vi "FF, Acceptance Criteria.vi"(8 "error in":errorcluster, 9 "n rows":i32=10, 10 "test case":T1, 11 "Tbl Refnum":refnum<vi>) -> (0 "error out":errorcluster, 3 "Tbl Refnum out":refnum<vi>)   [LabVIEW 2010]
doc: "This function transfers a single Compare Data Test (CDT) record to the current TestStand sequence step."
uses:
  Active Output Test Cases.ctl
panel:
  in  "Initialize Table":bool
  out "import error":errorcluster caption="error out"
  in  "Excel Clipboard to Import":string="TRS1763\tStimulus Phase Amplitude\t\t-5.170\t-4.830\tmA\tGELE\t%.3f\t%.3f\tTC1\nTRS1762\tStimulus Phase Pulse Width\t\t7.52\t16.48\tus\tGELE\t%.2f\t%.2f\tTC1\nTRS1761\tActive Interphase Delay\t\t13.0\t27.0\tus\tGELE\t%.1f\t%.1f\tTC1\nTRS1760\tActive Recovery Phase Amplitude\t\t4.830\t5.170\tmA\tGELE\t%.3f\t%.3f\tTC1\nTRS1759\tActive Recovery Phase Pulse Width\t\t7.5\t16.5\tus\tGELE\t%.1f\t%.1f\tTC1\nTRS1758\tFrequency\t\t1930.0\t2070.0\tHz\tGELE\t%.1f\t%.1f\tTC1\nTRS1757\tPulse Period Jitter (RMS)\t\t-2.500\t2.500\tus\tGELE\t%.1f\t%.1f\tTC1\nTRS1770\tStimulus Phase Amplitude\t\t-0.125\t0.085\tmA\tGELE\t%.3f\t%.3f\tTC2\nTRS1769\tStimulus Phase Pulse Width\t\t1436.0\t1564.0\tus\tGELE\t%.1f\t%.1f\tTC2\nTRS1768\tActive Interphase Delay\t\t233.0\t247.0\tus\tGELE\t%.1f\t%.1f\tTC2\nTRS1767\tActive Recovery Phase Amplitude\t\t-0.085\t0.125\tmA\tGELE\t%.3f\t%.3f\tTC2\nTRS1766\tActive Recovery Phase Pulse Width\t\t1436.0\t1564.0\tus\tGELE\t%.1f\t%.1f\tTC2\nTRS1765\tFrequency\t\t21.230\t22.770\tHz\tGELE\t%.3f\t%.3f\tTC2\nTRS1764\tPulse Period Jitter (RMS)\t\t-227.273\t227.273\tus\tGELE\t%.1f\t%.1f\tTC2\nTRS1777\tStimulus Phase Amplitude\t\t-15.320\t-14.680\tmA\tGELE\t%.3f\t%.3f\tTC3\nTRS1776\tStimulus Phase Pulse Width\t\t380.000\t420.000\tus\tGELE\t%.1f\t%.1f\tTC3\nTRS1775\tActive Interphase Delay\t\t93.0\t107.0\tus\tGELE\t%.1f\t%.1f\tTC3\nTRS1774\tActive Recovery Phase Amplitude\t\t14.680\t15.320\tmA\tGELE\t%.3f\t%.3f\tTC3\nTRS1773\tActive Recovery Phase Pulse Width\t\t380.00\t420.00\tus\tGELE\t%.1f\t%.1f\tTC3\nTRS1772\tFrequency\t\t1.930\t2.070\tHz\tGELE\t%.3f\t%.3f\tTC3\nTRS1771\tPulse Period Jitter (RMS)\t\t-2500.0\t2500.0\tus\tGELE\t%.1f\t%.1f\tTC3\nTRS1784\tStimulus Phase Amplitude\t\t2.850\t3.150\tmA\tGELE\t%.3f\t%.3f\tTC4\nTRS1783\tStimulus Phase Pulse Width\t\t1436.0\t1564.0\tus\tGELE\t%.1f\t%.1f\tTC4\nTRS1782\tActive Interphase Delay\t\t233.0\t247.0\tus\tGELE\t%.1f\t%.1f\tTC4\nTRS1781\tActive Recovery Phase Amplitude\t\t-0.726\t-0.474\tmA\tGELE\t%.3f\t%.3f\tTC4\nTRS1780\tActive Recovery Phase Pulse Width\t\t7180.0\t7820.0\tus\tGELE\t%.1f\t%.1f\tTC4\nTRS1779\tFrequency\t\t48.3\t51.8\tHz\tGELE\t%.1f\t%.1f\tTC4\nTRS1778\tPulse Period Jitter (RMS)\t\t-100.0\t100.0\tus\tGELE\t%.1f\t%.1f\tTC4\nTRS1791\tStimulus Phase Amplitude\t\t-0.085\t0.125\tmA\tGELE\t%.3f\t%.3f\tTC5\nTRS1790\tStimulus Phase Pulse Width\t\t1436.0\t1564.0\tus\tGELE\t%.1f\t%.1f\tTC5\nTRS1789\tActive Interphase Delay\t\t233.0\t247.0\tus\tGELE\t%.1f\t%.1f\tTC5\nTRS1788\tActive Recovery Phase Amplitude\t\t-0.125\t0.085\tmA\tGELE\t%.3f\t%.3f\tTC5\nTRS1787\tActive Recovery Phase Pulse Width\t\t1436.0\t1564.0\tus\tGELE\t%.1f\t%.1f\tTC5\nTRS1786\tFrequency\t\t21.230\t22.770\tHz\tGELE\t%.3f\t%.3f\tTC5\nTRS1785\tPulse Period Jitter (RMS)\t\t-227.3\t227.3\tus\tGELE\t%.1f\t%.1f\tTC5\nTRS1798\tStimulus Phase Amplitude\t\t14.680\t15.320\tmA\tGELE\t%.3f\t%.3f\tTC6\nTRS1797\tStimulus Phase Pulse Width\t\t380.0\t420.0\tus\tGELE\t%.1f\t%.1f\tTC6\nTRS1796\tActive Interphase Delay\t\t93.0\t107.0\tus\tGELE\t%.1f\t%.1f\tTC6\nTRS1795\tActive Recovery Phase Amplitude\t\t-15.320\t-14.680\tmA\tGELE\t%.3f\t%.3f\tTC6\nTRS1794\tActive Recovery Phase Pulse Width\t\t380.0\t420.0\tus\tGELE\t%.1f\t%.1f\tTC6\nTRS1793\tFrequency\t\t1.930\t2.070\tHz\tGELE\t%.3f\t%.3f\tTC6\nTRS1792\tPulse Period Jitter (RMS)\t\t-2500.0\t2500.0\tus\tGELE\t%.1f\t%.1f\tTC6\nTRS1805\tStimulus Phase Amplitude\t\t-5.170\t-4.830\tmA\tGELE\t%.3f\t%.3f\tTC7\nTRS1804\tStimulus Phase Pulse Width\t\t7.52\t16.48\tus\tGELE\t%.2f\t%.2f\tTC7\nTRS1803\tActive Interphase Delay\t\t13.0\t27.0\tus\tGELE\t%.1f\t%.1f\tTC7\nTRS1802\tActive Recovery Phase Amplitude\t\t4.830\t5.145\tmA\tGELE\t%.3f\t%.3f\tTC7\nTRS1801\tActive Recovery Phase Pulse Width\t\t7.5\t16.5\tus\tGELE\t%.1f\t%.1f\tTC7\nTRS1800\tFrequency\t\t1930.0\t2070.0\tHz\tGELE\t%.1f\t%.1f\tTC7\nTRS1799\tPulse Period Jitter (RMS)\t\t-2.5\t2.5\tus\tGELE\t%.1f\t%.1f\tTC7\nTRS1812\tStimulus Phase Amplitude\t\t-0.125\t0.085\tmA\tGELE\t%.3f\t%.3f\tTC8\nTRS1811\tStimulus Phase Pulse Width\t\t1436.0\t1564.0\tus\tGELE\t%.1f\t%.1f\tTC8\nTRS1810\tActive Interphase Delay\t\t233.0\t247.0\tus\tGELE\t%.1f\t%.1f\tTC8\nTRS1809\tActive Recovery Phase Amplitude\t\t-0.085\t0.125\tmA\tGELE\t%.3f\t%.3f\tTC8\nTRS1808\tActive Recovery Phase Pulse Width\t\t1436.0\t1564.0\tus\tGELE\t%.1f\t%.1f\tTC8\nTRS1807\tFrequency\t\t21.230\t22.770\tHz\tGELE\t%.3f\t%.3f\tTC8\nTRS1806\tPulse Period Jitter (RMS)\t\t-227.273\t227.273\tus\tGELE\t%.1f\t%.1f\tTC8\nTRS1819\tStimulus Phase Amplitude\t\t-30.620\t-29.380\tmA\tGELE\t%.3f\t%.3f\tTC9\nTRS1818\tStimulus Phase Pulse Width\t\t380.0\t420.0\tus\tGELE\t%.1f\t%.1f\tTC9\nTRS1817\tActive Interphase Delay\t\t93.0\t107.0\tus\tGELE\t%.1f\t%.1f\tTC9\nTRS1816\tActive Recovery Phase Amplitude\t\t29.380\t30.620\tmA\tGELE\t%.3f\t%.3f\tTC9\nTRS1815\tActive Recovery Phase Pulse Width\t\t380.0\t420.0\tus\tGELE\t%.1f\t%.1f\tTC9\nTRS1814\tFrequency\t\t1.930\t2.070\tHz\tGELE\t%.3f\t%.3f\tTC9\nTRS1813\tPulse Period Jitter (RMS)\t\t-2500.0\t2500.0\tus\tGELE\t%.1f\t%.1f\tTC9\nTRS1826\tStimulus Phase Amplitude\t\t2.850\t3.150\tmA\tGELE\t%.3f\t%.3f\tTC10\nTRS1825\tStimulus Phase Pulse Width\t\t1436.0\t1564.0\tus\tGELE\t%.1f\t%.1f\tTC10\nTRS1824\tActive Interphase Delay\t\t233.0\t247.0\tus\tGELE\t%.1f\t%.1f\tTC10\nTRS1823\tActive Recovery Phase Amplitude\t\t-0.726\t-0.474\tmA\tGELE\t%.3f\t%.3f\tTC10\nTRS1822\tActive Recovery Phase Pulse Width\t\t7180.0\t7820.0\tus\tGELE\t%.1f\t%.1f\tTC10\nTRS1821\tFrequency\t\t48.250\t51.750\tHz\tGELE\t%.1f\t%.1f\tTC10\nTRS1820\tPulse Period Jitter (RMS)\t\t-100.0\t100.0\tus\tGELE\t%.1f\t%.1f\tTC10\nTRS1833\tStimulus Phase Amplitude\t\t-0.085\t0.125\tmA\tGELE\t%.3f\t%.3f\tTC11\nTRS1832\tStimulus Phase Pulse Width\t\t1436.0\t1564.0\tus\tGELE\t%.1f\t%.1f\tTC11\nTRS1831\tActive Interphase Delay\t\t233.0\t247.0\tus\tGELE\t%.1f\t%.1f\tTC11\nTRS1830\tActive Recovery Phase Amplitude\t\t-0.125\t0.085\tmA\tGELE\t%.3f\t%.3f\tTC11\nTRS1829\tActive Recovery Phase Pulse Width\t\t1436.0\t1564.0\tus\tGELE\t%.1f\t%.1f\tTC11\nTRS1828\tFrequency\t\t21.230\t22.770\tHz\tGELE\t%.3f\t%.3f\tTC11\nTRS1827\tPulse Period Jitter (RMS)\t\t-227.3\t227.3\tus\tGELE\t%.1f\t%.1f\tTC11\nTRS1840\tStimulus Phase Amplitude\t\t29.380\t30.620\tmA\tGELE\t%.3f\t%.3f\tTC12\nTRS1839\tStimulus Phase Pulse Width\t\t380.0\t420.0\tus\tGELE\t%.1f\t%.1f\tTC12\nTRS1838\tActive Interphase Delay\t\t93.0\t107.0\tus\tGELE\t%.1f\t%.1f\tTC12\nTRS1837\tActive Recovery Phase Amplitude\t\t-30.620\t-29.380\tmA\tGELE\t%.3f\t%.3f\tTC12\nTRS1836\tActive Recovery Phase Pulse Width\t\t380.0\t420.0\tus\tGELE\t%.1f\t%.1f\tTC12\nTRS1835\tFrequency\t\t1.930\t2.070\tHz\tGELE\t%.3f\t%.3f\tTC12\nTRS1834\tPulse Period Jitter (RMS)\t\t-2500.0\t2500.0\tus\tGELE\t%.1f\t%.1f\tTC12\ntbd\tReserved\t\t\t\t\t\t\t\tTC13\ntbd\tReserved\t\t\t\t\t\t\t\tTC14\nTRS2009\tPulse 1,  Stimulus Phase Amplitude\t\t4.830\t5.170\tmA\tGELE\t%.3f\t%.3f\tTC15\nTRS2010\tPulse 2,  Stimulus Phase Amplitude\t\t3.840\t4.160\tmA\tGELE\t%.3f\t%.3f\tTC15\nTRS2011\tPulse 3,  Stimulus Phase Amplitude\t\t2.850\t3.150\tmA\tGELE\t%.3f\t%.3f\tTC15\nTRS2012\tPulse 4,  Stimulus Phase Amplitude\t\t1.860\t2.140\tmA\tGELE\t%.3f\t%.3f\tTC15\nTRS2013\tPulse 1,  Stimulus Phase Pulse  Width\t\t476.0\t524.0\tus\tGELE\t%.1f\t%.1f\tTC15\nTRS2014\tPulse 2,  Stimulus Phase Pulse  Width\t\t476.0\t524.0\tus\tGELE\t%.1f\t%.1f\tTC15\nTRS2015\tPulse 3,  Stimulus Phase Pulse  Width\t\t476.0\t524.0\tus\tGELE\t%.1f\t%.1f\tTC15\nTRS2016\tPulse 4,  Stimulus Phase Pulse  Width\t\t476.0\t524.0\tus\tGELE\t%.1f\t%.1f\tTC15\nTRS2017\tPulse 1,  Passive Interphase Delay\t\t118.0\t132.0\tus\tGELE\t%.1f\t%.1f\tTC15\nTRS2018\tPulse 2,  Passive Interphase Delay\t\t118.0\t132.0\tus\tGELE\t%.1f\t%.1f\tTC15\nTRS2019\tPulse 3,  Passive Interphase Delay\t\t118.0\t132.0\tus\tGELE\t%.1f\t%.1f\tTC15\nTRS2020\tPulse 4,  Passive Interphase Delay\t\t118.0\t132.0\tus\tGELE\t%.1f\t%.1f\tTC15\nTRS2021\tFrequency\t\t57.9\t62.1\tHz\tGELE\t%.3f\t%.3f\tTC15\nTRS2022\tPulse 1,  Stimulus Phase Amplitude\t\t4.830\t5.170\tmA\tGELE\t%.3f\t%.3f\tTC16\nTRS2023\tPulse 2,  Stimulus Phase Amplitude\t\t3.840\t4.160\tmA\tGELE\t%.3f\t%.3f\tTC16\nTRS2024\tPulse 3,  Stimulus Phase Amplitude\t\t2.850\t3.150\tmA\tGELE\t%.3f\t%.3f\tTC16\nTRS2025\tPulse 4,  Stimulus Phase Amplitude\t\t1.860\t2.140\tmA\tGELE\t%.3f\t%.3f\tTC16\nTRS2026\tPulse 1,  Stimulus Phase Pulse  Width\t\t476.0\t524.0\tus\tGELE\t%.1f\t%.1f\tTC16\nTRS2027\tPulse 2,  Stimulus Phase Pulse  Width\t\t476.0\t524.0\tus\tGELE\t%.1f\t%.1f\tTC16\nTRS2028\tPulse 3,  Stimulus Phase Pulse  Width\t\t476.0\t524.0\tus\tGELE\t%.1f\t%.1f\tTC16\nTRS2029\tPulse 4,  Stimulus Phase Pulse  Width\t\t476.0\t524.0\tus\tGELE\t%.1f\t%.1f\tTC16\nTRS2030\tPulse 1,  Active Interphase Delay\t\t143.0\t157.0\tus\tGELE\t%.1f\t%.1f\tTC16\nTRS2031\tPulse 2,  Active Interphase Delay\t\t143.0\t157.0\tus\tGELE\t%.1f\t%.1f\tTC16\nTRS2032\tPulse 3,  Active Interphase Delay\t\t143.0\t157.0\tus\tGELE\t%.1f\t%.1f\tTC16\nTRS2033\tPulse 4,  Active Interphase Delay\t\t143.0\t157.0\tus\tGELE\t%.1f\t%.1f\tTC16\nTRS2034\tPulse 1,  Active Recovery Phase Amplitude\t\t-1.130\t-0.890\tmA\tGELE\t%.3f\t%.3f\tTC16\nTRS2035\tPulse 2,  Active Recovery Phase Amplitude\t\t-0.928\t-0.688\tmA\tGELE\t%.3f\t%.3f\tTC16\nTRS2036\tPulse 3,  Active Recovery Phase Amplitude\t\t-0.726\t-0.486\tmA\tGELE\t%.3f\t%.3f\tTC16\nTRS2037\tPulse 4,  Active Recovery Phase Amplitude\t\t-0.524\t-0.284\tmA\tGELE\t%.3f\t%.3f\tTC16\nTRS2038\tPulse 1,  Active Recovery Phase Pulse  Width\t\t2380.0\t2620.0\tus\tGELE\t%.1f\t%.1f\tTC16\nTRS2039\tPulse 2,  Active Recovery Phase Pulse  Width\t\t2380.0\t2620.0\tus\tGELE\t%.1f\t%.1f\tTC16\nTRS2040\tPulse 3,  Active Recovery Phase Pulse  Width\t\t2380.0\t2620.0\tus\tGELE\t%.1f\t%.1f\tTC16\nTRS2041\tPulse 4,  Active Recovery Phase Pulse  Width\t\t2380.0\t2620.0\tus\tGELE\t%.1f\t%.1f\tTC16\nTRS2042\tFrequency\t\t62.725\t67.275\tHz\tGELE\t%.3f\t%.3f\tTC16\nTRS2043\tPulse 1,  Stimulus Phase Amplitude\t\t4.830\t5.170\tmA\tGELE\t%.3f\t%.3f\tTC17\nTRS2044\tPulse 2,  Stimulus Phase Amplitude\t\t3.840\t4.160\tmA\tGELE\t%.3f\t%.3f\tTC17\nTRS2045\tPulse 3,  Stimulus Phase Amplitude\t\t2.850\t3.150\tmA\tGELE\t%.3f\t%.3f\tTC17\nTRS2046\tPulse 4,  Stimulus Phase Amplitude\t\t1.860\t2.140\tmA\tGELE\t%.3f\t%.3f\tTC17\nTRS2047\tPulse 1,  Stimulus Phase Pulse  Width\t\t476.0\t524.0\tus\tGELE\t%.1f\t%.1f\tTC17\nTRS2048\tPulse 2,  Stimulus Phase Pulse  Width\t\t476.0\t524.0\tus\tGELE\t%.1f\t%.1f\tTC17\nTRS2049\tPulse 3,  Stimulus Phase Pulse  Width\t\t476.0\t524.0\tus\tGELE\t%.1f\t%.1f\tTC17\nTRS2050\tPulse 4,  Stimulus Phase Pulse  Width\t\t476.0\t524.0\tus\tGELE\t%.1f\t%.1f\tTC17\nTRS2051\tPulse 1,  Passive Interphase Delay\t\t118.0\t132.0\tus\tGELE\t%.1f\t%.1f\tTC17\nTRS2052\tPulse 2,  Passive Interphase Delay\t\t118.0\t132.0\tus\tGELE\t%.1f\t%.1f\tTC17\nTRS2053\tPulse 3,  Passive Interphase Delay\t\t118.0\t132.0\tus\tGELE\t%.1f\t%.1f\tTC17\nTRS2054\tPulse 4,  Passive Interphase Delay\t\t118.0\t132.0\tus\tGELE\t%.1f\t%.1f\tTC17\nTRS2055\tFrequency\t\t57.900\t62.100\tHz\tGELE\t%.3f\t%.3f\tTC17\nTRS1875\tStimulus Phase Amplitude\t\t14.680\t15.320\tmA\tGELE\t%.3f\t%.3f\tTC18\nTRS1876\tStimulus Phase Pulse Width\t\t284.0\t316.0\tus\tGELE\t%.1f\t%.1f\tTC18\nTRS1996\tActive Interphase Delay\t\t93.0\t107.0\tus\tGELE\t%.1f\t%.1f\tTC18\nTRS1997\tActive Recovery Phase Amplitude\t\t-15.320\t-14.680\tmA\tGELE\t%.3f\t%.3f\tTC18\nTRS1998\tActive Recovery Phase Pulse Width\t\t284.0\t316.0\tus\tGELE\t%.1f\t%.1f\tTC18\nTRS1877\tFrequency\t\t173.700\t186.300\tHz\tGELE\t%.3f\t%.3f\tTC18\nTRS1995\tPulse Period Jitter (RMS)\t\t-27.8\t27.8\tus\tGELE\t%.1f\t%.1f\tTC18\nTRS2135\tIPG Charging State\t\tCHARGE_CC_FAST-2\t\t-\tIgnoreCase\t-\t-\t\nTRS2136\tVBAT Voltage, Pre-Temp Stage 2\t\t3.75\t4.20\tV\tGELE\t%.2f\t%.2f\tTC19\nTRS2137\tIPG Temperature Level\t\t0\t2\t-\tGELE\t%.0f\t%.0f\tTC19\nTRS2138\tIPG Received Level\t\t6.00\t12.75\tV\tGELE\t%.2f\t%.2f\tTC19\nTRS2139\tCorrected IPG Temperature, Telemetry\t\t37.25\t37.75\t°C\tGELE\t%.2f\t%.2f\tTC19\nTRS2140\tAir Blast Temperature, RTD1\t\t35.25\t39.75\t°C\tGELE\t%.2f\t%.2f\tTC19\nTRS2141\tAir Blast Temperature, RTD2\t\t35.25\t39.75\t°C\tGELE\t%.2f\t%.2f\tTC19\nTRS2142\tTest Cartridge Temperature, RTD3\t\t35.0\t40.0\t°C\tGELE\t%.1f\t%.1f\tTC19\nTRS2143\tChamber Ambient Temperature, RTD4\t\t35.0\t40.0\t°C\tGELE\t%.1f\t%.1f\tTC19\nTRS2144\tIPG to RTD1 Temperature Offset\t\t-2.5\t2.5\t°C\tGELE\t%.1f\t%.1f\tTC19\nTRS2145\tVBAT Voltage, Post-Temp Stage 2\t\t3.75\t4.20\tV\tGELE\t%.2f\t%.2f\tTC19\nTRS2146\tIPG Charging State\t\tCHARGE_CC_FAST-2\t\t-\tIgnoreCase\t-\t-\t\nTRS2147\tVBAT Voltage, Pre-Temp Stage 3\t\t3.75\t4.20\tV\tGELE\t%.2f\t%.2f\tTC20\nTRS2148\tIPG Temperature Level\t\t0\t2\t-\tGELE\t%.0f\t%.0f\tTC20\nTRS2149\tIPG Received Level\t\t6.00\t12.75\tV\tGELE\t%.2f\t%.2f\tTC20\nTRS2150\tCorrected IPG Temperature, Telemetry\t\t40.0\t40.5\t°C\tGELE\t%.1f\t%.1f\tTC20\nTRS2151\tAir Blast Temperature, RTD1\t\t38.0\t42.5\t°C\tGELE\t%.1f\t%.1f\tTC20\nTRS2152\tAir Blast Temperature, RTD2\t\t38.0\t42.5\t°C\tGELE\t%.1f\t%.1f\tTC20\nTRS2153\tTest Cartridge Temperature, RTD3\t\t35.0\t40.0\t°C\tGELE\t%.1f\t%.1f\tTC20\nTRS2154\tChamber Ambient Temperature, RTD4\t\t35.0\t40.0\t°C\tGELE\t%.1f\t%.1f\tTC20\nTRS2155\tIPG to RTD1 Temperature Offset\t\t-2.5\t2.5\t°C\tGELE\t%.1f\t%.1f\tTC20\nTRS2156\tVBAT Voltage, Post-Temp Stage 3\t\t3.75\t4.20\tV\tGELE\t%.2f\t%.2f\tTC20\nTRS2157\tIPG Charging State\t\tCHARGE_CC_SLOW-3\t\t-\tIgnoreCase\t-\t-\t\nTRS2158\tVBAT Voltage, Pre-Temp Stage 4\t\t3.75\t4.20\tV\tGELE\t%.2f\t%.2f\tTC21\nTRS2159\tIPG Temperature Level\t\t3\t0\t-\tEQ\t%.0f\t%.0f\tTC21\nTRS2160\tIPG Received Level\t\t6.00\t12.75\tV\tGELE\t%.2f\t%.2f\tTC21\nTRS2161\tCorrected IPG Temperature, Telemetry\t\t41.0\t41.5\t°C\tGELE\t%.1f\t%.1f\tTC21\nTRS2162\tAir Blast Temperature, RTD1\t\t39.0\t43.5\t°C\tGELE\t%.1f\t%.1f\tTC21\nTRS2163\tAir Blast Temperature, RTD2\t\t39.0\t43.5\t°C\tGELE\t%.1f\t%.1f\tTC21\nTRS2164\tTest Cartridge Temperature, RTD3\t\t35.0\t40.0\t°C\tGELE\t%.1f\t%.1f\tTC21\nTRS2165\tChamber Ambient Temperature, RTD4\t\t35.0\t40.0\t°C\tGELE\t%.1f\t%.1f\tTC21\nTRS2166\tIPG to RTD1 Temperature Offset\t\t-2.5\t2.5\t°C\tGELE\t%.1f\t%.1f\tTC21\nTRS2167\tVBAT Voltage, Post-Temp Stage 4\t\t3.75\t4.20\tV\tGELE\t%.2f\t%.2f\tTC21\nTRS2168\tIPG Charging State\t\tCHARGE_OFF\t\t-\tIgnoreCase\t-\t-\t\nTRS2169\tVBAT Voltage, Pre-Temp Stage 5\t\t3.75\t4.20\tV\tGELE\t%.2f\t%.2f\tTC22\nTRS2170\tIPG Temperature Level\t\t4\t0\t-\tEQ\t%.0f\t%.0f\tTC22\nTRS2171\tIPG Received Level\t\t6.00\t12.75\tV\tGELE\t%.2f\t%.2f\tTC22\nTRS2172\tCorrected IPG Temperature, Telemetry\t\t42.0\t42.5\t°C\tGELE\t%.1f\t%.1f\tTC22\nTRS2173\tAir Blast Temperature, RTD1\t\t40.0\t44.5\t°C\tGELE\t%.1f\t%.1f\tTC22\nTRS2174\tAir Blast Temperature, RTD2\t\t40.0\t44.5\t°C\tGELE\t%.1f\t%.1f\tTC22\nTRS2175\tTest Cartridge Temperature, RTD3\t\t35.0\t40.0\t°C\tGELE\t%.1f\t%.1f\tTC22\nTRS2176\tChamber Ambient Temperature, RTD4\t\t35.0\t40.0\t°C\tGELE\t%.1f\t%.1f\tTC22\nTRS2177\tIPG to RTD1 Temperature Offset\t\t-2.5\t2.5\t°C\tGELE\t%.1f\t%.1f\tTC22\nTRS2178\tVBAT Voltage, Post-Temp Stage 5\t\t3.75\t4.20\tV\tGELE\t%.2f\t%.2f\tTC22\nTRS2179\tIPG Charging State\t\tCHARGE_OFF\t\t-\tIgnoreCase\t-\t-\t\nTRS2180\tVBAT Voltage, Pre-Temp Stage 6\t\t3.75\t4.20\tV\tGELE\t%.2f\t%.2f\tTC23\nTRS2181\tIPG Temperature Level\t\t0\t2\t-\tGELE\t%.0f\t%.0f\tTC23\nTRS2182\tIPG Received Level\t\t0.00\t1.20\tV\tGELE\t%.2f\t%.2f\tTC23\nTRS2183\tCorrected IPG Temperature, Telemetry\t\t35.75\t36.25\t°C\tGELE\t%.2f\t%.2f\tTC23\nTRS2184\tAir Blast Temperature, RTD1\t\t34.75\t37.25\t°C\tGELE\t%.2f\t%.2f\tTC23\nTRS2185\tAir Blast Temperature, RTD2\t\t34.75\t37.25\t°C\tGELE\t%.2f\t%.2f\tTC23\nTRS2186\tTest Cartridge Temperature, RTD3\t\t35.0\t40.0\t°C\tGELE\t%.1f\t%.1f\tTC23\nTRS2187\tChamber Ambient Temperature, RTD4\t\t35.0\t40.0\t°C\tGELE\t%.1f\t%.1f\tTC23\nTRS2188\tIPG to RTD1 Temperature Offset\t\t-1.5\t1.5\t°C\tGELE\t%.1f\t%.1f\tTC23\nTRS2189\tVBAT Voltage, Post-Temp Stage 6\t\t3.75\t4.20\tV\tGELE\t%.2f\t%.2f\tTC23\nTRS2190\tIPG Charging State\t\tCHARGE_CC_FAST-2\t\t-\tIgnoreCase\t-\t-\t\nTRS2191\tVBAT Voltage, Pre-Temp Stage 7\t\t3.75\t4.20\tV\tGELE\t%.2f\t%.2f\tTC24\nTRS2192\tIPG Temperature Level\t\t0\t2\t-\tGELE\t%.0f\t%.0f\tTC24\nTRS2193\tIPG Received Level\t\t6.00\t12.75\tV\tGELE\t%.2f\t%.2f\tTC24\nTRS2194\tCorrected IPG Temperature, Telemetry\t\t35.75\t36.25\t°C\tGELE\t%.2f\t%.2f\tTC24\nTRS2195\tAir Blast Temperature, RTD1\t\t33.75\t38.25\t°C\tGELE\t%.2f\t%.2f\tTC24\nTRS2196\tAir Blast Temperature, RTD2\t\t33.75\t38.25\t°C\tGELE\t%.2f\t%.2f\tTC24\nTRS2197\tTest Cartridge Temperature, RTD3\t\t35.0\t40.0\t°C\tGELE\t%.1f\t%.1f\tTC24\nTRS2198\tChamber Ambient Temperature, RTD4\t\t35.0\t40.0\t°C\tGELE\t%.1f\t%.1f\tTC24\nTRS2199\tIPG to RTD1 Temperature Offset\t\t-2.5\t2.5\t°C\tGELE\t%.1f\t%.1f\tTC24\nTRS2200\tVBAT Voltage, Post-Temp Stage 7\t\t3.75\t4.20\tV\tGELE\t%.2f\t%.2f\tTC24\nTBD\tMin Threshold\t\t9.50\t10.50\t°C\tGELE\t%.2f\t%.2f\tTC25\nTBD\tWarning Threshold\t\t39.50\t40.50\t°C\tGELE\t%.2f\t%.2f\tTC25\nTBD\tCritical Threshold\t\t40.50\t41.50\t°C\tGELE\t%.2f\t%.2f\tTC25\nTBD\tAbort Threshold\t\t41.50\t42.50\t°C\tGELE\t%.2f\t%.2f\tTC25\ntbd\tReserved\t\t\t\t\t\t\t\tTC26\n\tAmbient Temperature, Charge Off\t\t\t\t\t\t\t\t\nTBD\tIPG Charging State\t\tCHARGE_OFF\t\t-\tIgnoreCase\t-\t-\t\nTBD\tVBAT Voltage, Pre Ambient Conditions, Charge Off\t\t3.75\t4.20\tV\tGELE\t%.2f\t%.2f\tTC27\nTBD\tIPG Temperature Level\t\t0\t2\t-\tGELE\t%.0f\t%.0f\tTC27\nTBD\tIPG Received Level\t\t0.00\t1.20\tV\tGELE\t%.2f\t%.2f\tTC27\nTBD\tCorrected IPG Temperature, Ambient Charge Off\t\t35.0\t40.0\t°C\tGELE\t%.1f\t%.1f\tTC27\nTBD\tAir Blast Temperature, RTD1\t\t35.0\t40.0\t°C\tGELE\t%.1f\t%.1f\tTC27\nTBD\tAir Blast Temperature, RTD2\t\t35.0\t40.0\t°C\tGELE\t%.1f\t%.1f\tTC27\nTBD\tTest Cartridge Temperature, RTD3\t\t35.0\t40.0\t°C\tGELE\t%.1f\t%.1f\tTC27\nTBD\tChamber Ambient Temperature, RTD4\t\t35.0\t40.0\t°C\tGELE\t%.1f\t%.1f\tTC27\nTBD\tIPG to RTD1 Temperature Offset\t\t-1.0\t1.0\t°C\tGELE\t%.1f\t%.1f\tTC27\n\tAmbient Temperature, Charge On\t\t\t\t\t\t\t\t\nTBD\tIPG Charging State\t\tCHARGE_CC_FAST-2\t\t-\tIgnoreCase\t-\t-\t\nTBD\tIPG Temperature Level\t\t0\t2\t-\tGELE\t%.0f\t%.0f\tTC28\nTBD\tIPG Received Level\t\t6.00\t12.75\tV\tGELE\t%.2f\t%.2f\tTC28\nTBD\tCorrected IPG Temperature, Ambient Charge On\t\t35.0\t40.0\t°C\tGELE\t%.1f\t%.1f\tTC28\nTBD\tAir Blast Temperature, RTD1\t\t35.0\t40.0\t°C\tGELE\t%.1f\t%.1f\tTC28\nTBD\tAir Blast Temperature, RTD2\t\t35.0\t40.0\t°C\tGELE\t%.1f\t%.1f\tTC28\nTBD\tTest Cartridge Temperature, RTD3\t\t35.0\t40.0\t°C\tGELE\t%.1f\t%.1f\tTC28\nTBD\tChamber Ambient Temperature, RTD4\t\t35.0\t40.0\t°C\tGELE\t%.1f\t%.1f\tTC28\nTBD\tIPG to RTD1 Temperature Offset\t\t-2.5\t2.5\t°C\tGELE\t%.1f\t%.1f\tTC28\nTBD\tVBAT Voltage, Post Ambient Conditions, Charge On\t\t3.75\t4.20\tV\tGELE\t%.2f\t%.2f\tTC28\n\tCritical Temperature Transition, Charge On\t\t\t\t\t\t\t\t\nTBD\tIPG Charging State\t\tCHARGE_CC_SLOW-3\t\t-\tIgnoreCase\t-\t-\t\nTBD\tIPG Temperature Level\t\t2\t3\t-\tGELE\t%.0f\t%.0f\tTC29\nTBD\tIPG Received Level\t\t6.00\t12.75\tV\tGELE\t%.2f\t%.2f\tTC29\nTBD\tCorrected IPG Temperature, Critical Threshold\t\t40.4\t41.6\t°C\tGELE\t%.1f\t%.1f\tTC29\nTBD\tAir Blast Temperature, RTD1\t\t38.0\t44.0\t°C\tGELE\t%.1f\t%.1f\tTC29\nTBD\tAir Blast Temperature, RTD2\t\t38.0\t44.0\t°C\tGELE\t%.1f\t%.1f\tTC29\nTBD\tTest Cartridge Temperature, RTD3\t\t35.0\t40.0\t°C\tGELE\t%.1f\t%.1f\tTC29\nTBD\tChamber Ambient Temperature, RTD4\t\t35.0\t40.0\t°C\tGELE\t%.1f\t%.1f\tTC29\nTBD\tIPG to RTD1 Temperature Offset\t\t-2.0\t2.0\t°C\tGELE\t%.1f\t%.1f\tTC29\nTBD\tVBAT Voltage, Post Critical Temperature Transition\t\t3.75\t4.20\tV\tGELE\t%.2f\t%.2f\tTC29\n\tAbort Temperature Transition, Charge On\t\t\t\t\t\t\t\t\nTBD\tIPG Charging State\t\tCHARGE_OFF-0\t\t-\tIgnoreCase\t-\t-\t\nTBD\tIPG Temperature Level\t\t3\t4\t-\tGELE\t%.0f\t%.0f\tTC30\nTBD\tIPG Received Level\t\t6.00\t12.75\tV\tGELE\t%.2f\t%.2f\tTC30\nTBD\tCorrected IPG Temperature, Abort Threshold\t\t41.4\t42.6\t°C\tGELE\t%.1f\t%.1f\tTC30\nTBD\tAir Blast Temperature, RTD1\t\t39.0\t45.0\t°C\tGELE\t%.1f\t%.1f\tTC30\nTBD\tAir Blast Temperature, RTD2\t\t39.0\t45.0\t°C\tGELE\t%.1f\t%.1f\tTC30\nTBD\tTest Cartridge Temperature, RTD3\t\t35.0\t40.0\t°C\tGELE\t%.1f\t%.1f\tTC30\nTBD\tChamber Ambient Temperature, RTD4\t\t35.0\t40.0\t°C\tGELE\t%.1f\t%.1f\tTC30\nTBD\tIPG to RTD1 Temperature Offset\t\t-2.0\t2.0\t°C\tGELE\t%.1f\t%.1f\tTC30\nTBD\tVBAT Voltage, Post Abort Temperature Transition\t\t3.75\t4.20\tV\tGELE\t%.2f\t%.2f\tTC30\n\t\t\t\t\t\t\t\t\t\nTBD\tIPG Charging State\t\tCHARGE_CC_SLOW-3\t\t-\tIgnoreCase\t-\t-\t\nTBD\tIPG Temperature Level\t\t2\t3\t-\tGELE\t%.0f\t%.0f\tTC31\nTBD\tIPG Received Level\t\t6.00\t12.75\tV\tGELE\t%.2f\t%.2f\tTC31\nTBD\tCorrected IPG Temperature, Re-Enable Charging\t\t40.4\t41.6\t°C\tGELE\t%.1f\t%.1f\tTC31\nTBD\tAir Blast Temperature, RTD1\t\t38.0\t44.0\t°C\tGELE\t%.1f\t%.1f\tTC31\nTBD\tAir Blast Temperature, RTD2\t\t38.0\t44.0\t°C\tGELE\t%.1f\t%.1f\tTC31\nTBD\tTest Cartridge Temperature, RTD3\t\t35.0\t40.0\t°C\tGELE\t%.1f\t%.1f\tTC31\nTBD\tChamber Ambient Temperature, RTD4\t\t35.0\t40.0\t°C\tGELE\t%.1f\t%.1f\tTC31\nTBD\tIPG to RTD1 Temperature Offset\t\t-2.5\t2.5\t°C\tGELE\t%.1f\t%.1f\tTC31\nTBD\tVBAT Voltage, Post Re-Enable Charging Transition\t\t3.75\t4.20\tV\tGELE\t%.2f\t%.2f\tTC31\n\tNetDC Pre-Global-Gain-Adjustment\t\t\t\t\t\t\t\t\n\tPulse 1, Amplitude, Min\t\t14.000\t16.000\tmA\tGELE\t%.3f\t%.3f\tNetDC_P1\n\tPulse 1, Amplitude, Max\t\t14.000\t16.000\tmA\tGELE\t%.3f\t%.3f\tNetDC_P1\n\tPulse 1, Amplitude, Mean\t\t14.000\t16.000\tmA\tGELE\t%.3f\t%.3f\tNetDC_P1\n\tPulse 1, Offset, Mean Ratio\t\t0.950\t1.050\t\tGELE\t%.3f\t%.3f\tNetDC_P1\n\tPulse 2, Amplitude, Min\t\t9.000\t11.000\tmA\tGELE\t%.3f\t%.3f\tNetDC_P2\n\tPulse 2, Amplitude, Max\t\t9.000\t11.000\tmA\tGELE\t%.3f\t%.3f\tNetDC_P2\n\tPulse 2, Amplitude, Mean\t\t9.000\t11.000\tmA\tGELE\t%.3f\t%.3f\tNetDC_P2\n\tPulse 2, Offset, Mean Ratio\t\t0.950\t1.050\t\tGELE\t%.3f\t%.3f\tNetDC_P2\n\tPulse 3, Amplitude, Min\t\t4.500\t5.500\tmA\tGELE\t%.3f\t%.3f\tNetDC_P3\n\tPulse 3, Amplitude, Max\t\t4.500\t5.500\tmA\tGELE\t%.3f\t%.3f\tNetDC_P3\n\tPulse 3, Amplitude, Mean\t\t4.500\t5.500\tmA\tGELE\t%.3f\t%.3f\tNetDC_P3\n\tPulse 3, Offset, Mean Ratio\t\t0.950\t1.050\t\tGELE\t%.3f\t%.3f\tNetDC_P3\n\tPulse 4, Amplitude, Min\t\t1.800\t2.200\tmA\tGELE\t%.3f\t%.3f\tNetDC_P4\n\tPulse 4, Amplitude, Max\t\t1.800\t2.200\tmA\tGELE\t%.3f\t%.3f\tNetDC_P4\n\tPulse 4, Amplitude, Mean\t\t1.800\t2.200\tmA\tGELE\t%.3f\t%.3f\tNetDC_P4\n\tPulse 4, Offset, Mean Ratio\t\t0.950\t1.050\t\tGELE\t%.3f\t%.3f\tNetDC_P4\n"
  in  "Acceptance Criteria":string[][](table)=[["TRS1763", "Stimulus Phase Amplitude", "", "-5.200", "-4.810", "mA", "GELE", "%.3f", "%.3f", "TC1"], ["TRS1762", "Stimulus Phase Pulse Width", "", "92.00", "108.00", "us", "GELE", "%.2f", "%.2f", "TC1"], ["TRS1761", "Active Interphase Delay", "", "13.0", "27.0", "us", "GELE", "%.1f", "%.1f", "TC1"], ["TRS1760", "Active Recovery Phase Amplitude", "", "4.810", "5.200", "mA", "GELE", "%.3f", "%.3f", "TC1"], ["TRS1759", "Active Recovery Phase Pulse Width", "", "91.0", "109.0", "us", "GELE", "%.1f", "%.1f", "TC1"], ["TRS1758", "Frequency", "", "965.0", "1035.0", "Hz", "GELE", "%.1f", "%.1f", "TC1"], ["TRS1757", "Pulse Period Jitter (RMS)", "", "-2.500", "2.500", "us", "GELE", "%.1f", "%.1f", "TC1"], ["TRS1770", "Stimulus Phase Amplitude", "", "-0.125", "0.085", "mA", "GELE", "%.3f", "%.3f", "TC2"], ["TRS1769", "Stimulus Phase Pulse Width", "", "1436.0", "1564.0", "us", "GELE", "%.1f", "%.1f", "TC2"], ["TRS1768", "Active Interphase Delay", "", "233.0", "247.0", "us", "GELE", "%.1f", "%.1f", "TC2"], ["TRS1767", "Active Recovery Phase Amplitude", "", "-0.085", "0.125", "mA", "GELE", "%.3f", "%.3f", "TC2"], ["TRS1766", "Active Recovery Phase Pulse Width", "", "1436.0", "1564.0", "us", "GELE", "%.1f", "%.1f", "TC2"], ["TRS1765", "Frequency", "", "21.230", "22.770", "Hz", "GELE", "%.3f", "%.3f", "TC2"], ["TRS1764", "Pulse Period Jitter (RMS)", "", "-227.273", "227.273", "us", "GELE", "%.1f", "%.1f", "TC2"], ["TRS1777", "Stimulus Phase Amplitude", "", "-15.400", "-14.610", "mA", "GELE", "%.3f", "%.3f", "TC3"], ["TRS1776", "Stimulus Phase Pulse Width", "", "380.000", "420.000", "us", "GELE", "%.1f", "%.1f", "TC3"], ["TRS1775", "Active Interphase Delay", "", "93.0", "107.0", "us", "GELE", "%.1f", "%.1f", "TC3"], ["TRS1774", "Active Recovery Phase Amplitude", "", "14.610", "15.400", "mA", "GELE", "%.3f", "%.3f", "TC3"], ["TRS1773", "Active Recovery Phase Pulse Width", "", "380.00", "420.00", "us", "GELE", "%.1f", "%.1f", "TC3"], ["TRS1772", "Frequency", "", "1.930", "2.070", "Hz", "GELE", "%.3f", "%.3f", "TC3"], ["TRS1771", "Pulse Period Jitter (RMS)", "", "-2500.0", "2500.0", "us", "GELE", "%.1f", "%.1f", "TC3"], ["TRS1784", "Stimulus Phase Amplitude", "", "2.840", "3.170", "mA", "GELE", "%.3f", "%.3f", "TC4"], ["TRS1783", "Stimulus Phase Pulse Width", "", "1436.0", "1564.0", "us", "GELE", "%.1f", "%.1f", "TC4"], ["TRS1782", "Active Interphase Delay", "", "233.0", "247.0", "us", "GELE", "%.1f", "%.1f", "TC4"], ["TRS1781", "Active Recovery Phase Amplitude", "", "-0.726", "-0.474", "mA", "GELE", "%.3f", "%.3f", "TC4"], ["TRS1780", "Active Recovery Phase Pulse Width", "", "7180.0", "7820.0", "us", "GELE", "%.1f", "%.1f", "TC4"], ["TRS1779", "Frequency", "", "48.3", "51.8", "Hz", "GELE", "%.1f", "%.1f", "TC4"], ["TRS1778", "Pulse Period Jitter (RMS)", "", "-100.0", "100.0", "us", "GELE", "%.1f", "%.1f", "TC4"], ["TRS1791", "Stimulus Phase Amplitude", "", "-0.085", "0.125", "mA", "GELE", "%.3f", "%.3f", "TC5"], ["TRS1790", "Stimulus Phase Pulse Width", "", "1436.0", "1564.0", "us", "GELE", "%.1f", "%.1f", "TC5"], ["TRS1789", "Active Interphase Delay", "", "233.0", "247.0", "us", "GELE", "%.1f", "%.1f", "TC5"], ["TRS1788", "Active Recovery Phase Amplitude", "", "-0.125", "0.085", "mA", "GELE", "%.3f", "%.3f", "TC5"], ["TRS1787", "Active Recovery Phase Pulse Width", "", "1436.0", "1564.0", "us", "GELE", "%.1f", "%.1f", "TC5"], ["TRS1786", "Frequency", "", "21.230", "22.770", "Hz", "GELE", "%.3f", "%.3f", "TC5"], ["TRS1785", "Pulse Period Jitter (RMS)", "", "-227.3", "227.3", "us", "GELE", "%.1f", "%.1f", "TC5"], ["TRS1798", "Stimulus Phase Amplitude", "", "14.610", "15.400", "mA", "GELE", "%.3f", "%.3f", "TC6"], ["TRS1797", "Stimulus Phase Pulse Width", "", "380.0", "420.0", "us", "GELE", "%.1f", "%.1f", "TC6"], ["TRS1796", "Active Interphase Delay", "", "93.0", "107.0", "us", "GELE", "%.1f", "%.1f", "TC6"], ["TRS1795", "Active Recovery Phase Amplitude", "", "-15.400", "-14.610", "mA", "GELE", "%.3f", "%.3f", "TC6"], ["TRS1794", "Active Recovery Phase Pulse Width", "", "380.0", "420.0", "us", "GELE", "%.1f", "%.1f", "TC6"], ["TRS1793", "Frequency", "", "1.930", "2.070", "Hz", "GELE", "%.3f", "%.3f", "TC6"], ["TRS1792", "Pulse Period Jitter (RMS)", "", "-2500.0", "2500.0", "us", "GELE", "%.1f", "%.1f", "TC6"], ["TRS1805", "Stimulus Phase Amplitude", "", "-5.200", "-4.810", "mA", "GELE", "%.3f", "%.3f", "TC7"], ["TRS1804", "Stimulus Phase Pulse Width", "", "92.00", "108.00", "us", "GELE", "%.2f", "%.2f", "TC7"], ["TRS1803", "Active Interphase Delay", "", "13.0", "27.0", "us", "GELE", "%.1f", "%.1f", "TC7"], ["TRS1802", "Active Recovery Phase Amplitude", "", "4.810", "5.170", "mA", "GELE", "%.3f", "%.3f", "TC7"], ["TRS1801", "Active Recovery Phase Pulse Width", "", "91.0", "109.0", "us", "GELE", "%.1f", "%.1f", "TC7"], ["TRS1800", "Frequency", "", "965.0", "1035.0", "Hz", "GELE", "%.1f", "%.1f", "TC7"], ["TRS1799", "Pulse Period Jitter (RMS)", "", "-2.5", "2.5", "us", "GELE", "%.1f", "%.1f", "TC7"], ["TRS1812", "Stimulus Phase Amplitude", "", "-0.125", "0.085", "mA", "GELE", "%.3f", "%.3f", "TC8"], ["TRS1811", "Stimulus Phase Pulse Width", "", "1436.0", "1564.0", "us", "GELE", "%.1f", "%.1f", "TC8"], ["TRS1810", "Active Interphase Delay", "", "233.0", "247.0", "us", "GELE", "%.1f", "%.1f", "TC8"], ["TRS1809", "Active Recovery Phase Amplitude", "", "-0.085", "0.125", "mA", "GELE", "%.3f", "%.3f", "TC8"], ["TRS1808", "Active Recovery Phase Pulse Width", "", "1436.0", "1564.0", "us", "GELE", "%.1f", "%.1f", "TC8"], ["TRS1807", "Frequency", "", "21.230", "22.770", "Hz", "GELE", "%.3f", "%.3f", "TC8"], ["TRS1806", "Pulse Period Jitter (RMS)", "", "-227.273", "227.273", "us", "GELE", "%.1f", "%.1f", "TC8"], ["TRS1819", "Stimulus Phase Amplitude", "", "-30.770", "-29.230", "mA", "GELE", "%.3f", "%.3f", "TC9"], ["TRS1818", "Stimulus Phase Pulse Width", "", "380.0", "420.0", "us", "GELE", "%.1f", "%.1f", "TC9"], ["TRS1817", "Active Interphase Delay", "", "93.0", "107.0", "us", "GELE", "%.1f", "%.1f", "TC9"], ["TRS1816", "Active Recovery Phase Amplitude", "", "29.230", "30.770", "mA", "GELE", "%.3f", "%.3f", "TC9"], ["TRS1815", "Active Recovery Phase Pulse Width", "", "380.0", "420.0", "us", "GELE", "%.1f", "%.1f", "TC9"], ["TRS1814", "Frequency", "", "1.930", "2.070", "Hz", "GELE", "%.3f", "%.3f", "TC9"], ["TRS1813", "Pulse Period Jitter (RMS)", "", "-2500.0", "2500.0", "us", "GELE", "%.1f", "%.1f", "TC9"], ["TRS1826", "Stimulus Phase Amplitude", "", "2.840", "3.170", "mA", "GELE", "%.3f", "%.3f", "TC10"], ["TRS1825", "Stimulus Phase Pulse Width", "", "1436.0", "1564.0", "us", "GELE", "%.1f", "%.1f", "TC10"], ["TRS1824", "Active Interphase Delay", "", "233.0", "247.0", "us", "GELE", "%.1f", "%.1f", "TC10"], ["TRS1823", "Active Recovery Phase Amplitude", "", "-0.726", "-0.474", "mA", "GELE", "%.3f", "%.3f", "TC10"], ["TRS1822", "Active Recovery Phase Pulse Width", "", "7180.0", "7820.0", "us", "GELE", "%.1f", "%.1f", "TC10"], ["TRS1821", "Frequency", "", "48.250", "51.750", "Hz", "GELE", "%.1f", "%.1f", "TC10"], ["TRS1820", "Pulse Period Jitter (RMS)", "", "-100.0", "100.0", "us", "GELE", "%.1f", "%.1f", "TC10"], ["TRS1833", "Stimulus Phase Amplitude", "", "-0.085", "0.125", "mA", "GELE", "%.3f", "%.3f", "TC11"], ["TRS1832", "Stimulus Phase Pulse Width", "", "1436.0", "1564.0", "us", "GELE", "%.1f", "%.1f", "TC11"], ["TRS1831", "Active Interphase Delay", "", "233.0", "247.0", "us", "GELE", "%.1f", "%.1f", "TC11"], ["TRS1830", "Active Recovery Phase Amplitude", "", "-0.125", "0.085", "mA", "GELE", "%.3f", "%.3f", "TC11"], ["TRS1829", "Active Recovery Phase Pulse Width", "", "1436.0", "1564.0", "us", "GELE", "%.1f", "%.1f", "TC11"], ["TRS1828", "Frequency", "", "21.230", "22.770", "Hz", "GELE", "%.3f", "%.3f", "TC11"], ["TRS1827", "Pulse Period Jitter (RMS)", "", "-227.3", "227.3", "us", "GELE", "%.1f", "%.1f", "TC11"], ["TRS1840", "Stimulus Phase Amplitude", "", "29.230", "30.770", "mA", "GELE", "%.3f", "%.3f", "TC12"], ["TRS1839", "Stimulus Phase Pulse Width", "", "380.0", "420.0", "us", "GELE", "%.1f", "%.1f", "TC12"], ["TRS1838", "Active Interphase Delay", "", "93.0", "107.0", "us", "GELE", "%.1f", "%.1f", "TC12"], ["TRS1837", "Active Recovery Phase Amplitude", "", "-30.770", "-29.230", "mA", "GELE", "%.3f", "%.3f", "TC12"], ["TRS1836", "Active Recovery Phase Pulse Width", "", "380.0", "420.0", "us", "GELE", "%.1f", "%.1f", "TC12"], ["TRS1835", "Frequency", "", "1.930", "2.070", "Hz", "GELE", "%.3f", "%.3f", "TC12"], ["TRS1834", "Pulse Period Jitter (RMS)", "", "-2500.0", "2500.0", "us", "GELE", "%.1f", "%.1f", "TC12"], ["tbd", "Reserved", "", "", "", "", "", "", "", "TC13"], ["tbd", "Reserved", "", "", "", "", "", "", "", "TC14"], ["TRS2009", "Pulse 1,  Stimulus Phase Amplitude", "", "4.830", "5.170", "mA", "GELE", "%.3f", "%.3f", "TC15"], ["TRS2010", "Pulse 2,  Stimulus Phase Amplitude", "", "3.840", "4.160", "mA", "GELE", "%.3f", "%.3f", "TC15"], ["TRS2011", "Pulse 3,  Stimulus Phase Amplitude", "", "2.850", "3.150", "mA", "GELE", "%.3f", "%.3f", "TC15"], ["TRS2012", "Pulse 4,  Stimulus Phase Amplitude", "", "1.860", "2.140", "mA", "GELE", "%.3f", "%.3f", "TC15"], ["TRS2013", "Pulse 1,  Stimulus Phase Pulse  Width", "", "476.0", "524.0", "us", "GELE", "%.1f", "%.1f", "TC15"], ["TRS2014", "Pulse 2,  Stimulus Phase Pulse  Width", "", "476.0", "524.0", "us", "GELE", "%.1f", "%.1f", "TC15"], ["TRS2015", "Pulse 3,  Stimulus Phase Pulse  Width", "", "476.0", "524.0", "us", "GELE", "%.1f", "%.1f", "TC15"], ["TRS2016", "Pulse 4,  Stimulus Phase Pulse  Width", "", "476.0", "524.0", "us", "GELE", "%.1f", "%.1f", "TC15"], ["TRS2017", "Pulse 1,  Passive Interphase Delay", "", "118.0", "132.0", "us", "GELE", "%.1f", "%.1f", "TC15"], ["TRS2018", "Pulse 2,  Passive Interphase Delay", "", "118.0", "132.0", "us", "GELE", "%.1f", "%.1f", "TC15"], ["TRS2019", "Pulse 3,  Passive Interphase Delay", "", "118.0", "132.0", "us", "GELE", "%.1f", "%.1f", "TC15"], ["TRS2020", "Pulse 4,  Passive Interphase Delay", "", "118.0", "132.0", "us", "GELE", "%.1f", "%.1f", "TC15"], ["TRS2021", "Frequency", "", "57.9", "62.1", "Hz", "GELE", "%.3f", "%.3f", "TC15"], ["TRS2022", "Pulse 1,  Stimulus Phase Amplitude", "", "4.830", "5.170", "mA", "GELE", "%.3f", "%.3f", "TC16"], ["TRS2023", "Pulse 2,  Stimulus Phase Amplitude", "", "3.840", "4.160", "mA", "GELE", "%.3f", "%.3f", "TC16"], ["TRS2024", "Pulse 3,  Stimulus Phase Amplitude", "", "2.850", "3.150", "mA", "GELE", "%.3f", "%.3f", "TC16"], ["TRS2025", "Pulse 4,  Stimulus Phase Amplitude", "", "1.860", "2.140", "mA", "GELE", "%.3f", "%.3f", "TC16"], ["TRS2026", "Pulse 1,  Stimulus Phase Pulse  Width", "", "476.0", "524.0", "us", "GELE", "%.1f", "%.1f", "TC16"], ["TRS2027", "Pulse 2,  Stimulus Phase Pulse  Width", "", "476.0", "524.0", "us", "GELE", "%.1f", "%.1f", "TC16"], ["TRS2028", "Pulse 3,  Stimulus Phase Pulse  Width", "", "476.0", "524.0", "us", "GELE", "%.1f", "%.1f", "TC16"], ["TRS2029", "Pulse 4,  Stimulus Phase Pulse  Width", "", "476.0", "524.0", "us", "GELE", "%.1f", "%.1f", "TC16"], ["TRS2030", "Pulse 1,  Active Interphase Delay", "", "143.0", "157.0", "us", "GELE", "%.1f", "%.1f", "TC16"], ["TRS2031", "Pulse 2,  Active Interphase Delay", "", "143.0", "157.0", "us", "GELE", "%.1f", "%.1f", "TC16"], ["TRS2032", "Pulse 3,  Active Interphase Delay", "", "143.0", "157.0", "us", "GELE", "%.1f", "%.1f", "TC16"], ["TRS2033", "Pulse 4,  Active Interphase Delay", "", "143.0", "157.0", "us", "GELE", "%.1f", "%.1f", "TC16"], ["TRS2034", "Pulse 1,  Active Recovery Phase Amplitude", "", "-1.130", "-0.890", "mA", "GELE", "%.3f", "%.3f", "TC16"], ["TRS2035", "Pulse 2,  Active Recovery Phase Amplitude", "", "-0.928", "-0.688", "mA", "GELE", "%.3f", "%.3f", "TC16"], ["TRS2036", "Pulse 3,  Active Recovery Phase Amplitude", "", "-0.726", "-0.486", "mA", "GELE", "%.3f", "%.3f", "TC16"], ["TRS2037", "Pulse 4,  Active Recovery Phase Amplitude", "", "-0.524", "-0.284", "mA", "GELE", "%.3f", "%.3f", "TC16"], ["TRS2038", "Pulse 1,  Active Recovery Phase Pulse  Width", "", "2380.0", "2620.0", "us", "GELE", "%.1f", "%.1f", "TC16"], ["TRS2039", "Pulse 2,  Active Recovery Phase Pulse  Width", "", "2380.0", "2620.0", "us", "GELE", "%.1f", "%.1f", "TC16"], ["TRS2040", "Pulse 3,  Active Recovery Phase Pulse  Width", "", "2380.0", "2620.0", "us", "GELE", "%.1f", "%.1f", "TC16"], ["TRS2041", "Pulse 4,  Active Recovery Phase Pulse  Width", "", "2380.0", "2620.0", "us", "GELE", "%.1f", "%.1f", "TC16"], ["TRS2042", "Frequency", "", "62.725", "67.275", "Hz", "GELE", "%.3f", "%.3f", "TC16"], ["TRS2043", "Pulse 1,  Stimulus Phase Amplitude", "", "4.830", "5.170", "mA", "GELE", "%.3f", "%.3f", "TC17"], ["TRS2044", "Pulse 2,  Stimulus Phase Amplitude", "", "3.840", "4.160", "mA", "GELE", "%.3f", "%.3f", "TC17"], ["TRS2045", "Pulse 3,  Stimulus Phase Amplitude", "", "2.850", "3.150", "mA", "GELE", "%.3f", "%.3f", "TC17"], ["TRS2046", "Pulse 4,  Stimulus Phase Amplitude", "", "1.860", "2.140", "mA", "GELE", "%.3f", "%.3f", "TC17"], ["TRS2047", "Pulse 1,  Stimulus Phase Pulse  Width", "", "476.0", "524.0", "us", "GELE", "%.1f", "%.1f", "TC17"], ["TRS2048", "Pulse 2,  Stimulus Phase Pulse  Width", "", "476.0", "524.0", "us", "GELE", "%.1f", "%.1f", "TC17"], ["TRS2049", "Pulse 3,  Stimulus Phase Pulse  Width", "", "476.0", "524.0", "us", "GELE", "%.1f", "%.1f", "TC17"], ["TRS2050", "Pulse 4,  Stimulus Phase Pulse  Width", "", "476.0", "524.0", "us", "GELE", "%.1f", "%.1f", "TC17"], ["TRS2051", "Pulse 1,  Passive Interphase Delay", "", "118.0", "132.0", "us", "GELE", "%.1f", "%.1f", "TC17"], ["TRS2052", "Pulse 2,  Passive Interphase Delay", "", "118.0", "132.0", "us", "GELE", "%.1f", "%.1f", "TC17"], ["TRS2053", "Pulse 3,  Passive Interphase Delay", "", "118.0", "132.0", "us", "GELE", "%.1f", "%.1f", "TC17"], ["TRS2054", "Pulse 4,  Passive Interphase Delay", "", "118.0", "132.0", "us", "GELE", "%.1f", "%.1f", "TC17"], ["TRS2055", "Frequency", "", "57.900", "62.100", "Hz", "GELE", "%.3f", "%.3f", "TC17"], ["TRS1875", "Stimulus Phase Amplitude", "", "14.610", "15.400", "mA", "GELE", "%.3f", "%.3f", "TC18"], ["TRS1876", "Stimulus Phase Pulse Width", "", "284.0", "316.0", "us", "GELE", "%.1f", "%.1f", "TC18"], ["TRS1996", "Active Interphase Delay", "", "93.0", "107.0", "us", "GELE", "%.1f", "%.1f", "TC18"], ["TRS1997", "Active Recovery Phase Amplitude", "", "-15.400", "-14.610", "mA", "GELE", "%.3f", "%.3f", "TC18"], ["TRS1998", "Active Recovery Phase Pulse Width", "", "284.0", "316.0", "us", "GELE", "%.1f", "%.1f", "TC18"], ["TRS1877", "Frequency", "", "173.700", "186.300", "Hz", "GELE", "%.3f", "%.3f", "TC18"], ["TRS1995", "Pulse Period Jitter (RMS)", "", "-27.8", "27.8", "us", "GELE", "%.1f", "%.1f", "TC18"], ["TRS2135", "IPG Charging State", "", "CHARGE_CC_FAST-2", "", "-", "IgnoreCase", "-", "-", ""], ["TRS2136", "VBAT Voltage, Pre-Temp Stage 2", "", "3.75", "4.20", "V", "GELE", "%.2f", "%.2f", "TC19"], ["TRS2137", "IPG Temperature Level", "", "0", "2", "-", "GELE", "%.0f", "%.0f", "TC19"], ["TRS2138", "IPG Received Level", "", "6.00", "12.75", "V", "GELE", "%.2f", "%.2f", "TC19"], ["TRS2139", "Corrected IPG Temperature, Telemetry", "", "37.25", "37.75", "°C", "GELE", "%.2f", "%.2f", "TC19"], ["TRS2140", "Air Blast Temperature, RTD1", "", "35.25", "39.75", "°C", "GELE", "%.2f", "%.2f", "TC19"], ["TRS2141", "Air Blast Temperature, RTD2", "", "35.25", "39.75", "°C", "GELE", "%.2f", "%.2f", "TC19"], ["TRS2142", "Test Cartridge Temperature, RTD3", "", "35.0", "40.0", "°C", "GELE", "%.1f", "%.1f", "TC19"], ["TRS2143", "Chamber Ambient Temperature, RTD4", "", "35.0", "40.0", "°C", "GELE", "%.1f", "%.1f", "TC19"], ["TRS2144", "IPG to RTD1 Temperature Offset", "", "-2.5", "2.5", "°C", "GELE", "%.1f", "%.1f", "TC19"], ["TRS2145", "VBAT Voltage, Post-Temp Stage 2", "", "3.75", "4.20", "V", "GELE", "%.2f", "%.2f", "TC19"], ["TRS2146", "IPG Charging State", "", "CHARGE_CC_FAST-2", "", "-", "IgnoreCase", "-", "-", ""], ["TRS2147", "VBAT Voltage, Pre-Temp Stage 3", "", "3.75", "4.20", "V", "GELE", "%.2f", "%.2f", "TC20"], ["TRS2148", "IPG Temperature Level", "", "0", "2", "-", "GELE", "%.0f", "%.0f", "TC20"], ["TRS2149", "IPG Received Level", "", "6.00", "12.75", "V", "GELE", "%.2f", "%.2f", "TC20"], ["TRS2150", "Corrected IPG Temperature, Telemetry", "", "40.0", "40.5", "°C", "GELE", "%.1f", "%.1f", "TC20"], ["TRS2151", "Air Blast Temperature, RTD1", "", "38.0", "42.5", "°C", "GELE", "%.1f", "%.1f", "TC20"], ["TRS2152", "Air Blast Temperature, RTD2", "", "38.0", "42.5", "°C", "GELE", "%.1f", "%.1f", "TC20"], ["TRS2153", "Test Cartridge Temperature, RTD3", "", "35.0", "40.0", "°C", "GELE", "%.1f", "%.1f", "TC20"], ["TRS2154", "Chamber Ambient Temperature, RTD4", "", "35.0", "40.0", "°C", "GELE", "%.1f", "%.1f", "TC20"], ["TRS2155", "IPG to RTD1 Temperature Offset", "", "-2.5", "2.5", "°C", "GELE", "%.1f", "%.1f", "TC20"], ["TRS2156", "VBAT Voltage, Post-Temp Stage 3", "", "3.75", "4.20", "V", "GELE", "%.2f", "%.2f", "TC20"], ["TRS2157", "IPG Charging State", "", "CHARGE_CC_SLOW-3", "", "-", "IgnoreCase", "-", "-", ""], ["TRS2158", "VBAT Voltage, Pre-Temp Stage 4", "", "3.75", "4.20", "V", "GELE", "%.2f", "%.2f", "TC21"], ["TRS2159", "IPG Temperature Level", "", "3", "0", "-", "EQ", "%.0f", "%.0f", "TC21"], ["TRS2160", "IPG Received Level", "", "6.00", "12.75", "V", "GELE", "%.2f", "%.2f", "TC21"], ["TRS2161", "Corrected IPG Temperature, Telemetry", "", "41.0", "41.5", "°C", "GELE", "%.1f", "%.1f", "TC21"], ["TRS2162", "Air Blast Temperature, RTD1", "", "39.0", "43.5", "°C", "GELE", "%.1f", "%.1f", "TC21"], ["TRS2163", "Air Blast Temperature, RTD2", "", "39.0", "43.5", "°C", "GELE", "%.1f", "%.1f", "TC21"], ["TRS2164", "Test Cartridge Temperature, RTD3", "", "35.0", "40.0", "°C", "GELE", "%.1f", "%.1f", "TC21"], ["TRS2165", "Chamber Ambient Temperature, RTD4", "", "35.0", "40.0", "°C", "GELE", "%.1f", "%.1f", "TC21"], ["TRS2166", "IPG to RTD1 Temperature Offset", "", "-2.5", "2.5", "°C", "GELE", "%.1f", "%.1f", "TC21"], ["TRS2167", "VBAT Voltage, Post-Temp Stage 4", "", "3.75", "4.20", "V", "GELE", "%.2f", "%.2f", "TC21"], ["TRS2168", "IPG Charging State", "", "CHARGE_OFF", "", "-", "IgnoreCase", "-", "-", ""], ["TRS2169", "VBAT Voltage, Pre-Temp Stage 5", "", "3.75", "4.20", "V", "GELE", "%.2f", "%.2f", "TC22"], ["TRS2170", "IPG Temperature Level", "", "4", "0", "-", "EQ", "%.0f", "%.0f", "TC22"], ["TRS2171", "IPG Received Level", "", "6.00", "12.75", "V", "GELE", "%.2f", "%.2f", "TC22"], ["TRS2172", "Corrected IPG Temperature, Telemetry", "", "42.0", "42.5", "°C", "GELE", "%.1f", "%.1f", "TC22"], ["TRS2173", "Air Blast Temperature, RTD1", "", "40.0", "44.5", "°C", "GELE", "%.1f", "%.1f", "TC22"], ["TRS2174", "Air Blast Temperature, RTD2", "", "40.0", "44.5", "°C", "GELE", "%.1f", "%.1f", "TC22"], ["TRS2175", "Test Cartridge Temperature, RTD3", "", "35.0", "40.0", "°C", "GELE", "%.1f", "%.1f", "TC22"], ["TRS2176", "Chamber Ambient Temperature, RTD4", "", "35.0", "40.0", "°C", "GELE", "%.1f", "%.1f", "TC22"], ["TRS2177", "IPG to RTD1 Temperature Offset", "", "-2.5", "2.5", "°C", "GELE", "%.1f", "%.1f", "TC22"], ["TRS2178", "VBAT Voltage, Post-Temp Stage 5", "", "3.75", "4.20", "V", "GELE", "%.2f", "%.2f", "TC22"], ["TRS2179", "IPG Charging State", "", "CHARGE_OFF", "", "-", "IgnoreCase", "-", "-", ""], ["TRS2180", "VBAT Voltage, Pre-Temp Stage 6", "", "3.75", "4.20", "V", "GELE", "%.2f", "%.2f", "TC23"], ["TRS2181", "IPG Temperature Level", "", "0", "2", "-", "GELE", "%.0f", "%.0f", "TC23"], ["TRS2182", "IPG Received Level", "", "0.00", "1.20", "V", "GELE", "%.2f", "%.2f", "TC23"], ["TRS2183", "Corrected IPG Temperature, Telemetry", "", "35.75", "36.25", "°C", "GELE", "%.2f", "%.2f", "TC23"], ["TRS2184", "Air Blast Temperature, RTD1", "", "34.75", "37.25", "°C", "GELE", "%.2f", "%.2f", "TC23"], ["TRS2185", "Air Blast Temperature, RTD2", "", "34.75", "37.25", "°C", "GELE", "%.2f", "%.2f", "TC23"], ["TRS2186", "Test Cartridge Temperature, RTD3", "", "35.0", "40.0", "°C", "GELE", "%.1f", "%.1f", "TC23"], ["TRS2187", "Chamber Ambient Temperature, RTD4", "", "35.0", "40.0", "°C", "GELE", "%.1f", "%.1f", "TC23"], ["TRS2188", "IPG to RTD1 Temperature Offset", "", "-1.5", "1.5", "°C", "GELE", "%.1f", "%.1f", "TC23"], ["TRS2189", "VBAT Voltage, Post-Temp Stage 6", "", "3.75", "4.20", "V", "GELE", "%.2f", "%.2f", "TC23"], ["TRS2190", "IPG Charging State", "", "CHARGE_CC_FAST-2", "", "-", "IgnoreCase", "-", "-", ""], ["TRS2191", "VBAT Voltage, Pre-Temp Stage 7", "", "3.75", "4.20", "V", "GELE", "%.2f", "%.2f", "TC24"], ["TRS2192", "IPG Temperature Level", "", "0", "2", "-", "GELE", "%.0f", "%.0f", "TC24"], ["TRS2193", "IPG Received Level", "", "6.00", "12.75", "V", "GELE", "%.2f", "%.2f", "TC24"], ["TRS2194", "Corrected IPG Temperature, Telemetry", "", "35.75", "36.25", "°C", "GELE", "%.2f", "%.2f", "TC24"], ["TRS2195", "Air Blast Temperature, RTD1", "", "33.75", "38.25", "°C", "GELE", "%.2f", "%.2f", "TC24"], ["TRS2196", "Air Blast Temperature, RTD2", "", "33.75", "38.25", "°C", "GELE", "%.2f", "%.2f", "TC24"], ["TRS2197", "Test Cartridge Temperature, RTD3", "", "35.0", "40.0", "°C", "GELE", "%.1f", "%.1f", "TC24"], ["TRS2198", "Chamber Ambient Temperature, RTD4", "", "35.0", "40.0", "°C", "GELE", "%.1f", "%.1f", "TC24"], ["TRS2199", "IPG to RTD1 Temperature Offset", "", "-2.5", "2.5", "°C", "GELE", "%.1f", "%.1f", "TC24"], ["TRS2200", "VBAT Voltage, Post-Temp Stage 7", "", "3.75", "4.20", "V", "GELE", "%.2f", "%.2f", "TC24"], ["TBD", "Min Threshold", "", "9.50", "10.50", "°C", "GELE", "%.2f", "%.2f", "TC25"], ["TBD", "Warning Threshold", "", "39.50", "40.50", "°C", "GELE", "%.2f", "%.2f", "TC25"], ["TBD", "Critical Threshold", "", "40.50", "41.50", "°C", "GELE", "%.2f", "%.2f", "TC25"], ["TBD", "Abort Threshold", "", "41.50", "42.50", "°C", "GELE", "%.2f", "%.2f", "TC25"], ["tbd", "Reserved", "", "", "", "", "", "", "", "TC26"], ["", "Ambient Temperature, Charge Off", "", "", "", "", "", "", "", ""], ["TBD", "IPG Charging State", "", "CHARGE_OFF", "", "-", "IgnoreCase", "-", "-", ""], ["TBD", "VBAT Voltage, Pre Ambient Conditions, Charge Off", "", "3.75", "4.20", "V", "GELE", "%.2f", "%.2f", "TC27"], ["TBD", "IPG Temperature Level", "", "0", "2", "-", "GELE", "%.0f", "%.0f", "TC27"], ["TBD", "IPG Received Level", "", "0.00", "1.20", "V", "GELE", "%.2f", "%.2f", "TC27"], ["TBD", "Corrected IPG Temperature, Ambient Charge Off", "", "35.0", "40.0", "°C", "GELE", "%.1f", "%.1f", "TC27"], ["TBD", "Air Blast Temperature, RTD1", "", "35.0", "40.0", "°C", "GELE", "%.1f", "%.1f", "TC27"], ["TBD", "Air Blast Temperature, RTD2", "", "35.0", "40.0", "°C", "GELE", "%.1f", "%.1f", "TC27"], ["TBD", "Test Cartridge Temperature, RTD3", "", "35.0", "40.0", "°C", "GELE", "%.1f", "%.1f", "TC27"], ["TBD", "Chamber Ambient Temperature, RTD4", "", "35.0", "40.0", "°C", "GELE", "%.1f", "%.1f", "TC27"], ["TBD", "IPG to RTD1 Temperature Offset", "", "-1.0", "1.0", "°C", "GELE", "%.1f", "%.1f", "TC27"], ["", "Ambient Temperature, Charge On", "", "", "", "", "", "", "", ""], ["TBD", "IPG Charging State", "", "CHARGE_CC_FAST-2", "", "-", "IgnoreCase", "-", "-", ""], ["TBD", "IPG Temperature Level", "", "0", "2", "-", "GELE", "%.0f", "%.0f", "TC28"], ["TBD", "IPG Received Level", "", "6.00", "12.75", "V", "GELE", "%.2f", "%.2f", "TC28"], ["TBD", "Corrected IPG Temperature, Ambient Charge On", "", "35.0", "40.0", "°C", "GELE", "%.1f", "%.1f", "TC28"], ["TBD", "Air Blast Temperature, RTD1", "", "35.0", "40.0", "°C", "GELE", "%.1f", "%.1f", "TC28"], ["TBD", "Air Blast Temperature, RTD2", "", "35.0", "40.0", "°C", "GELE", "%.1f", "%.1f", "TC28"], ["TBD", "Test Cartridge Temperature, RTD3", "", "35.0", "40.0", "°C", "GELE", "%.1f", "%.1f", "TC28"], ["TBD", "Chamber Ambient Temperature, RTD4", "", "35.0", "40.0", "°C", "GELE", "%.1f", "%.1f", "TC28"], ["TBD", "IPG to RTD1 Temperature Offset", "", "-2.5", "2.5", "°C", "GELE", "%.1f", "%.1f", "TC28"], ["TBD", "VBAT Voltage, Post Ambient Conditions, Charge On", "", "3.75", "4.20", "V", "GELE", "%.2f", "%.2f", "TC28"], ["", "Critical Temperature Transition, Charge On", "", "", "", "", "", "", "", ""], ["TBD", "IPG Charging State", "", "CHARGE_CC_SLOW-3", "", "-", "IgnoreCase", "-", "-", ""], ["TBD", "IPG Temperature Level", "", "2", "3", "-", "GELE", "%.0f", "%.0f", "TC29"], ["TBD", "IPG Received Level", "", "6.00", "12.75", "V", "GELE", "%.2f", "%.2f", "TC29"], ["TBD", "Corrected IPG Temperature, Critical Threshold", "", "40.0", "42.0", "°C", "GELE", "%.1f", "%.1f", "TC29"], ["TBD", "Air Blast Temperature, RTD1", "", "38.0", "44.0", "°C", "GELE", "%.1f", "%.1f", "TC29"], ["TBD", "Air Blast Temperature, RTD2", "", "38.0", "44.0", "°C", "GELE", "%.1f", "%.1f", "TC29"], ["TBD", "Test Cartridge Temperature, RTD3", "", "35.0", "40.0", "°C", "GELE", "%.1f", "%.1f", "TC29"], ["TBD", "Chamber Ambient Temperature, RTD4", "", "35.0", "40.0", "°C", "GELE", "%.1f", "%.1f", "TC29"], ["TBD", "IPG to RTD1 Temperature Offset", "", "-2.0", "2.0", "°C", "GELE", "%.1f", "%.1f", "TC29"], ["TBD", "VBAT Voltage, Post Critical Temperature Transition", "", "3.75", "4.20", "V", "GELE", "%.2f", "%.2f", "TC29"], ["", "Abort Temperature Transition, Charge On", "", "", "", "", "", "", "", ""], ["TBD", "IPG Charging State", "", "CHARGE_OFF-0", "", "-", "IgnoreCase", "-", "-", ""], ["TBD", "IPG Temperature Level", "", "3", "4", "-", "GELE", "%.0f", "%.0f", "TC30"], ["TBD", "IPG Received Level", "", "6.00", "12.75", "V", "GELE", "%.2f", "%.2f", "TC30"], ["TBD", "Corrected IPG Temperature, Abort Threshold", "", "41.0", "43.0", "°C", "GELE", "%.1f", "%.1f", "TC30"], ["TBD", "Air Blast Temperature, RTD1", "", "39.0", "45.0", "°C", "GELE", "%.1f", "%.1f", "TC30"], ["TBD", "Air Blast Temperature, RTD2", "", "39.0", "45.0", "°C", "GELE", "%.1f", "%.1f", "TC30"], ["TBD", "Test Cartridge Temperature, RTD3", "", "35.0", "40.0", "°C", "GELE", "%.1f", "%.1f", "TC30"], ["TBD", "Chamber Ambient Temperature, RTD4", "", "35.0", "40.0", "°C", "GELE", "%.1f", "%.1f", "TC30"], ["TBD", "IPG to RTD1 Temperature Offset", "", "-2.0", "2.0", "°C", "GELE", "%.1f", "%.1f", "TC30"], ["TBD", "VBAT Voltage, Post Abort Temperature Transition", "", "3.75", "4.20", "V", "GELE", "%.2f", "%.2f", "TC30"], ["", "", "", "", "", "", "", "", "", ""], ["TBD", "IPG Charging State", "", "CHARGE_CC_SLOW-3", "", "-", "IgnoreCase", "-", "-", ""], ["TBD", "IPG Temperature Level", "", "2", "3", "-", "GELE", "%.0f", "%.0f", "TC31"], ["TBD", "IPG Received Level", "", "6.00", "12.75", "V", "GELE", "%.2f", "%.2f", "TC31"], ["TBD", "Corrected IPG Temperature, Re-Enable Charging", "", "39.0", "42.0", "°C", "GELE", "%.1f", "%.1f", "TC31"], ["TBD", "Air Blast Temperature, RTD1", "", "38.0", "44.0", "°C", "GELE", "%.1f", "%.1f", "TC31"], ["TBD", "Air Blast Temperature, RTD2", "", "38.0", "44.0", "°C", "GELE", "%.1f", "%.1f", "TC31"], ["TBD", "Test Cartridge Temperature, RTD3", "", "35.0", "40.0", "°C", "GELE", "%.1f", "%.1f", "TC31"], ["TBD", "Chamber Ambient Temperature, RTD4", "", "35.0", "40.0", "°C", "GELE", "%.1f", "%.1f", "TC31"], ["TBD", "IPG to RTD1 Temperature Offset", "", "-2.5", "2.5", "°C", "GELE", "%.1f", "%.1f", "TC31"], ["TBD", "VBAT Voltage, Post Re-Enable Charging Transition", "", "3.75", "4.20", "V", "GELE", "%.2f", "%.2f", "TC31"], ["", "NetDC Pre-Global-Gain-Adjustment", "", "", "", "", "", "", "", ""], ["", "Pulse 1, Amplitude, Min", "", "14.000", "16.000", "mA", "GELE", "%.3f", "%.3f", "NetDC_P1"], ["", "Pulse 1, Amplitude, Max", "", "14.000", "16.000", "mA", "GELE", "%.3f", "%.3f", "NetDC_P1"], ["", "Pulse 1, Amplitude, Mean", "", "14.000", "16.000", "mA", "GELE", "%.3f", "%.3f", "NetDC_P1"], ["", "Pulse 1, Offset, Mean Ratio", "", "0.950", "1.050", "", "GELE", "%.3f", "%.3f", "NetDC_P1"], ["", "Pulse 2, Amplitude, Min", "", "9.000", "11.000", "mA", "GELE", "%.3f", "%.3f", "NetDC_P2"], ["", "Pulse 2, Amplitude, Max", "", "9.000", "11.000", "mA", "GELE", "%.3f", "%.3f", "NetDC_P2"], ["", "Pulse 2, Amplitude, Mean", "", "9.000", "11.000", "mA", "GELE", "%.3f", "%.3f", "NetDC_P2"], ["", "Pulse 2, Offset, Mean Ratio", "", "0.950", "1.050", "", "GELE", "%.3f", "%.3f", "NetDC_P2"], ["", "Pulse 3, Amplitude, Min", "", "4.500", "5.500", "mA", "GELE", "%.3f", "%.3f", "NetDC_P3"], ["", "Pulse 3, Amplitude, Max", "", "4.500", "5.500", "mA", "GELE", "%.3f", "%.3f", "NetDC_P3"], ["", "Pulse 3, Amplitude, Mean", "", "4.500", "5.500", "mA", "GELE", "%.3f", "%.3f", "NetDC_P3"], ["", "Pulse 3, Offset, Mean Ratio", "", "0.950", "1.050", "", "GELE", "%.3f", "%.3f", "NetDC_P3"], ["", "Pulse 4, Amplitude, Min", "", "1.800", "2.200", "mA", "GELE", "%.3f", "%.3f", "NetDC_P4"], ["", "Pulse 4, Amplitude, Max", "", "1.800", "2.200", "mA", "GELE", "%.3f", "%.3f", "NetDC_P4"], ["", "Pulse 4, Amplitude, Mean", "", "1.800", "2.200", "mA", "GELE", "%.3f", "%.3f", "NetDC_P4"], ["", "Pulse 4, Offset, Mean Ratio", "", "0.950", "1.050", "", "GELE", "%.3f", "%.3f", "NetDC_P4"]] caption="Table 1"
  # "(See instructions\non Block Diagram.)"
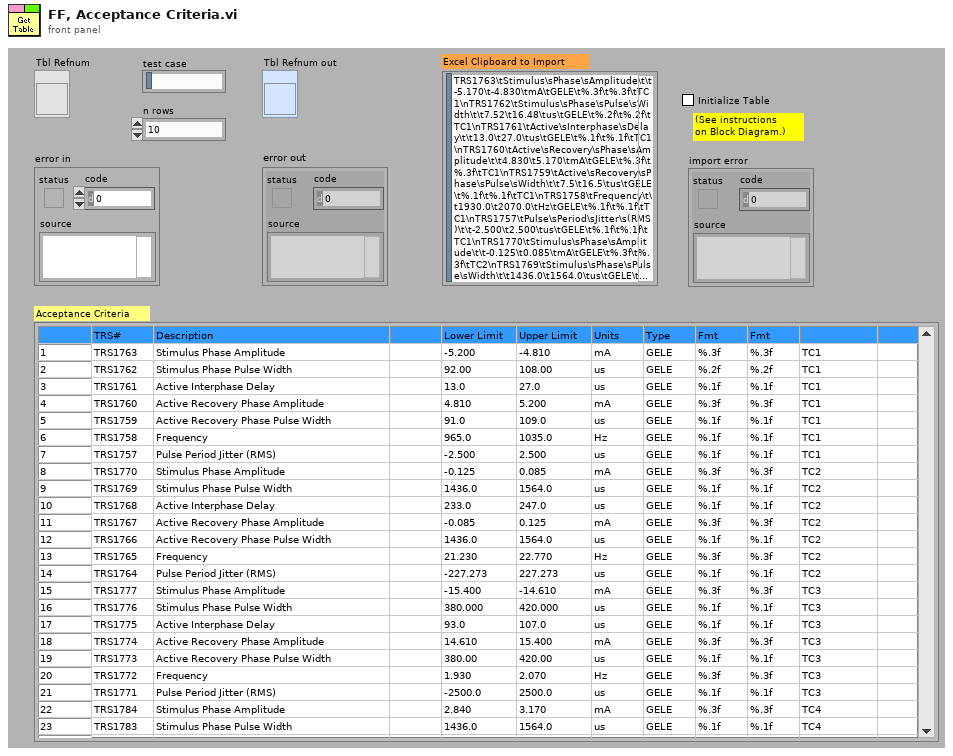
[diagram p1: front panel]
types:
  T1 = typedef "Active Output Test Cases.ctl" = string
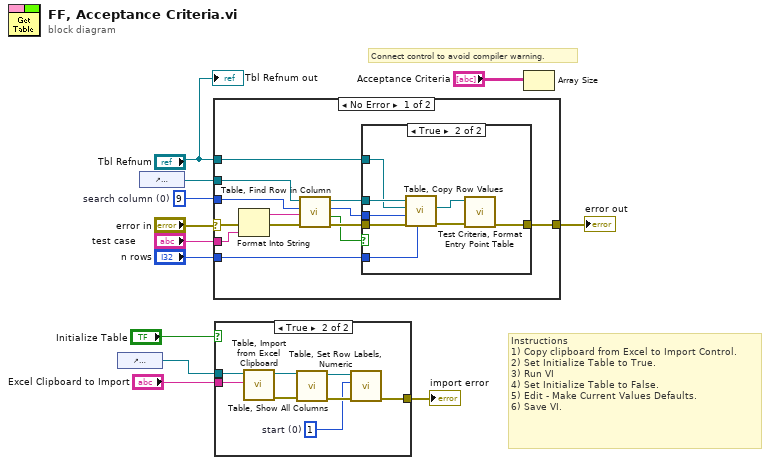
[diagram p0: block diagram]
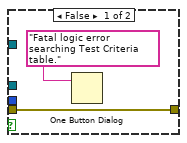
[diagram p3: hidden frame]
diagram:
  w1 = 9  # search column (0)
  # "Instructions\n1) Copy clipboard from Excel to Import Control.\n2) Set Initialize Table to True.\n3) Run VI \n4) Set Initialize Table to False.\n5) Edit - Make Current Values Defaults.\n6) Save VI."
  # "Connect control to avoid compiler warning."
  n1 = control-ref of="Acceptance Criteria"() -> (w6:refnum<vi>)
  n2 = control-ref of="Acceptance Criteria"() -> (w8:refnum<vi>)
  n3 = case shown="No Error" "error in" {
    selector: "error in" -> [w23 w36]
    tunnel: [w18 w36] -> w12
    tunnel: "test case" -> [w22 _]
    tunnel: "Tbl Refnum" -> [w19 _]
    tunnel: w8 -> [w16 _]
    tunnel: "n rows" -> [w15 _]
    tunnel: w1 -> [w14 _]
    frame No Error {
      n4 = Format Into String(error in=w23, w22) -> (resulting string=w25:string, error out=w24:errorcluster)  [unwired: 2 in]
      n5 = call "Table, Find Row in Column.vi"("error in"=w24, "search key"=w25, "search column (0)"=w14, "Tbl Refnum"=w16) -> ("error out"=w20:errorcluster, "found"=w17:bool, "row index"=w13:i32, "Tbl Refnum out"=w21:refnum<vi>)  [unwired: 4 in]
      n6 = case shown="True" w17 {
        tunnel: w21 -> [_ w34]
        tunnel: w20 -> [w27 w30]
        tunnel: [w27 w35] -> w18
        tunnel: w19 -> [_ w33]
        tunnel: w15 -> [_ w29]
        tunnel: w13 -> [_ w28]
        frame False {
          n7 = One Button Dialog(message="Fatal logic error searching Test Criteria table.") -> ()  [unwired: 1 in, 1 out]
        }
        frame True {
          n8 = call "Table, Copy Row Values.vi"("n rows (1)"=w29, "error in"=w30, "row (0)"=w28, "Tbl Refnum Dst"=w33, "Tbl Refnum Src"=w34) -> ("error out"=w31:errorcluster, "Tbl Refnum Dst out"=w32:refnum<vi>)  [unwired: 2 in, 1 out]
          n9 = call "Test Criteria, Format Entry Point Table.vi"("error in"=w31, "Tbl Refnum"=w32) -> ("error out"=w35:errorcluster)  [unwired: 8 in, 1 out]
        }
      }
    }
    frame Error {
    }
  }
  "error out" <- w12
  n10 = case shown="True" "Initialize Table" {
    tunnel: "Excel Clipboard to Import" -> [_ w39]
    tunnel: w6 -> [_ w38]
    tunnel: [_ w37] -> w5
    frame False {
    }
    frame True {
      w40 = 1  # start (0)
      n11 = call "Table, Import from Excel Clipboard.vi"("Excel Clipboard to Import"=w39, "Tbl Refnum"=w38) -> ("error out"=w43:errorcluster, "Tbl Refnumout"=w44:refnum<vi>)  [unwired: 8 in]
      n12 = call "Table, Show All Columns.vi"("error in"=w43, "Tbl Refnum"=w44) -> ("error out"=w42:errorcluster, "Tbl Refnum out"=w41:refnum<vi>)  [unwired: 8 in]
      n13 = call "Table, Set Row Labels, Numeric.vi"("error in"=w42, "start (0)"=w40, "Tbl Refnum"=w41) -> ("error out"=w37:errorcluster)  [unwired: 7 in, 1 out]
    }
  }
  "import error" <- w5
  n14 = Array Size(array="Acceptance Criteria") -> ()  [unwired: 1 out]
  "Tbl Refnum out" <- "Tbl Refnum"
